vi "Email_or_SMS.vi"(0 "Email address":string[](array[string])=["SMS to Mobile:p.hayden@surrey.ac.uk"]) -> (1 "Send Code":u32, 2 "Email":string[](array[string]), 3 "SMS to send":string[](array[string]), 4 "All Mobile Numbers":string[](array[string]))   [LabVIEW 2010]
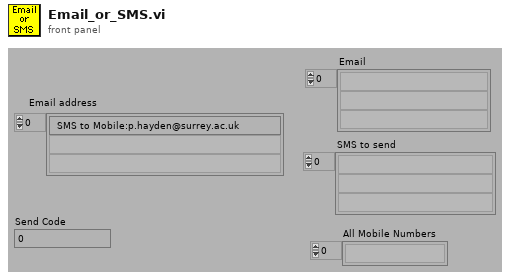
[diagram p1: front panel]
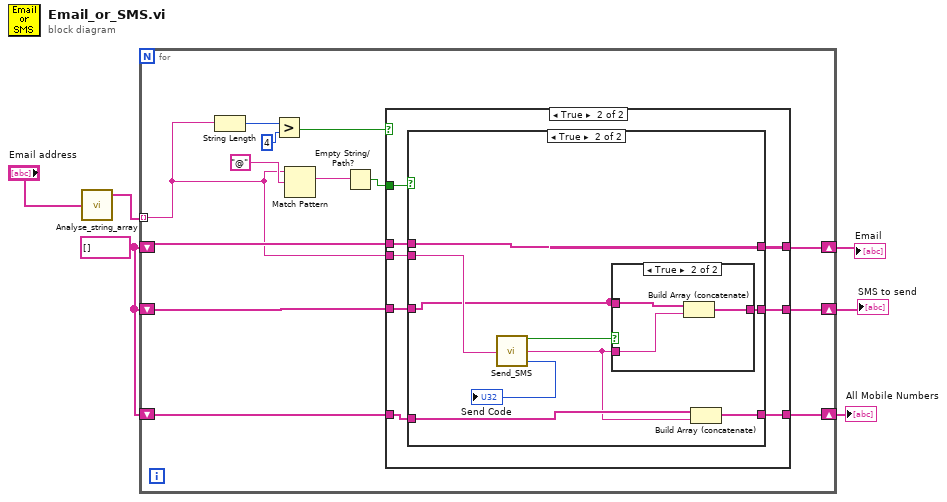
[diagram p0: block diagram]
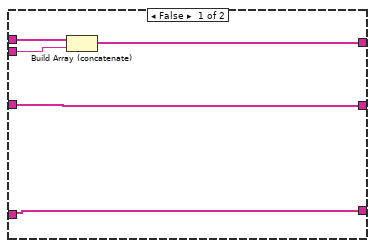
[diagram p3: hidden frame]
diagram:
  w4 = string[] []
  n1 = call "Analyse_string_array.vi"("String array"="Email address") -> ("Unique strings"=w6:string[])  [unwired: 2 out]
  n2 = for {
    tunnel: w6 -> [w10] mode=indexing
    shift-right: [w17] -> w5
    shift-left: w4 -> [w18]
    shift-right: [w16] -> w1
    shift-left: w4 -> [w15]
    shift-right: [w7] -> w3
    shift-left: w4 -> [w8]
    n3 = String Length(string=w10) -> (length=w14:i32)
    n4 = Greater?(x=w14, y=4) -> (0:w12:bool)
    n5 = Match Pattern(string=w10, regular expression="@") -> (match substring=w9:string)  [unwired: 4 out]
    n6 = Empty String/Path?(string/path=w9) -> (empty?=w19:bool)
    n7 = case shown="True" w12 {
      tunnel: w19 -> [_ w30]
      tunnel: w18 -> [w22 w29]
      tunnel: [w22 w28] -> w17
      tunnel: [w21 w27] -> w16
      tunnel: w15 -> [w21 w26]
      tunnel: w10 -> [_ w25]
      tunnel: w8 -> [w20 w24]
      tunnel: [w20 w23] -> w7
      frame False {
      }
      frame True {
        n8 = case shown="True" w30 {
          tunnel: w29 -> [w35 w43]
          tunnel: w25 -> [w34 w42]
          tunnel: [w33 w43] -> w28
          tunnel: [w32 w44] -> w27
          tunnel: w26 -> [w32 w40]
          tunnel: w24 -> [w31 w38]
          tunnel: [w31 w36] -> w23
          frame False {
            n9 = Build Array (concatenate)(w35, w34) -> (w33:string[])
          }
          frame True {
            n10 = call "Send_SMS.vi"("Mobile Number and code"=w42) -> ("Send?"=w41:bool, "Mobile Number"=w37:string, "Send Code"=→"Send Code":u32)
            n11 = case shown="True" w41 {
              tunnel: w40 -> [_ w48]
              tunnel: [w45 w47] -> w44
              tunnel: w37 -> [_ w46]
              tunnel: w40 -> [w45 _]
              frame False {
              }
              frame True {
                n12 = Build Array (concatenate)(w48, w46) -> (w47:string[])
              }
            }
            n13 = Build Array (concatenate)(w38, w37) -> (w36:string[])
          }
        }
      }
    }
  }
  "SMS to send" <- w1
  "Email" <- w5
  "All Mobile Numbers" <- w3
